vi "Read Data from Text File.vi"(9 "File Name (default: input.txt)":string="input.txt", 11 "Subfolder":string) -> (2 "data":string)   [LabVIEW 2021]
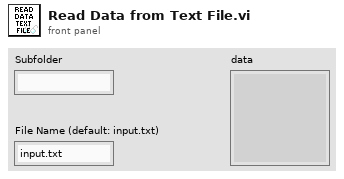
[diagram p1: front panel]
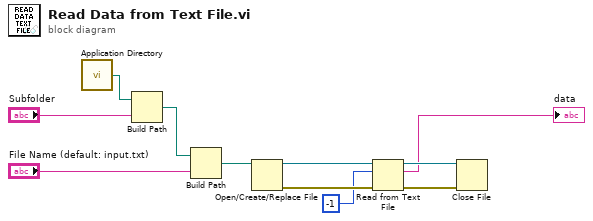
[diagram p0: block diagram]
diagram:
  n1 = call <vilib>:"Application Directory.vi"() -> ("Application Directory"=w4:path)
  n2 = Build Path(base path=w4, name or relative path="Subfolder") -> (appended path=w5:path)
  n3 = Build Path(base path=w5, name or relative path="File Name (default: input.txt)") -> (appended path=w2:path)
  n4 = Open/Create/Replace File(file path (use dialog)=w2) -> (refnum out=w11:refnum<file>, error out=w10:errorcluster)  [unwired: 5 in, 1 out]
  n5 = Read from Text File(file (use dialog)=w11, count=-1, error in=w10) -> (refnum out=w9:refnum<file>, text=→"data":string, error out=w8:errorcluster)  [unwired: 1 in, 1 out]
  n6 = Close File(refnum=w9, error in=w8) -> ()  [unwired: 2 out]
